vi "Find New Corners.vi"(0 "Updated Map":T1, 1 "Point":cluster{"Col":i16, "Row":i16}, 2 "# safety grids":i32=4) -> (5 "Corners":cluster{"Col":i16, "Row":i16}[](array[cluster]))   [LabVIEW 2009]
uses:
  <vilib>/Analysis/Matrix/Datatypes/RealMatrix.ctl
  <vilib>/Analysis/Matrix/NI_Matrix.lvlib
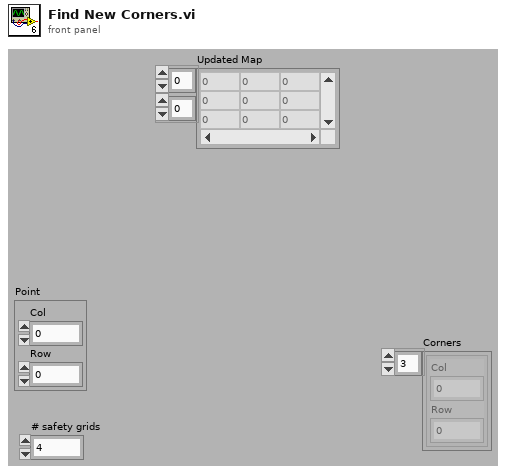
[diagram p1: front panel]
types:
  T1 = typedef "NI_Matrix.lvlib/RealMatrix.ctl" = dbl[][]
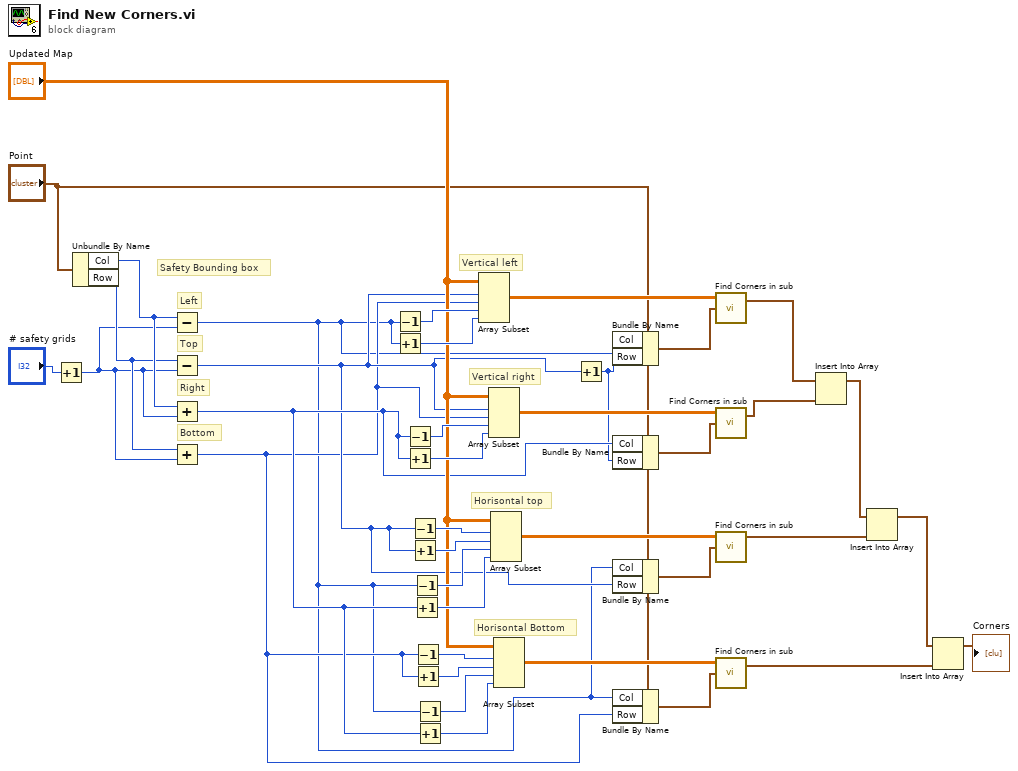
[diagram p0: block diagram]
diagram:
  # "Horisontal Bottom"
  # "Horisontal top"
  # "Vertical right"
  # "Vertical left"
  # "Safety Bounding box"
  # "Bottom"
  # "Top"
  # "Right"
  # "Left"
  n1 = Increment(x="# safety grids") -> (x+1=w2:i32)
  n2 = Unbundle By Name("Point") -> ("Col"=w38:i16, "Row"=w37:i16)
  n3 = Subtract(x=w38, y=w2) -> (x-y=w10:i32)
  n4 = Subtract(x=w37, y=w2) -> (x-y=w12:i32)
  n5 = Add(x=w38, y=w2) -> (x+y=w14:i32)
  n6 = Add(x=w37, y=w2) -> (x+y=w11:i32)
  n7 = Decrement(x=w10) -> (x-1=w36:i32)
  n8 = Increment(x=w10) -> (x+1=w35:i32)
  n9 = Decrement(x=w14) -> (x-1=w33:i32)
  n10 = Increment(x=w14) -> (x+1=w32:i32)
  n11 = Decrement(x=w12) -> (x-1=w29:i32)
  n12 = Increment(x=w12) -> (x+1=w28:i32)
  n13 = Decrement(x=w10) -> (x-1=w27:i32)
  n14 = Increment(x=w14) -> (x+1=w26:i32)
  n15 = Decrement(x=w11) -> (x-1=w24:i32)
  n16 = Increment(x=w11) -> (x+1=w23:i32)
  n17 = Decrement(x=w10) -> (x-1=w22:i32)
  n18 = Increment(x=w14) -> (x+1=w21:i32)
  n19 = Array Subset(array="Updated Map", index (row)=w12, length (row)=w11, index (col)=w36, length (col)=w35) -> (w34:T1)
  n20 = Array Subset(array="Updated Map", index (row)=w12, length (row)=w11, index (col)=w33, length (col)=w32) -> (w31:T1)
  n21 = Array Subset(array="Updated Map", index (row)=w29, length (row)=w28, index (col)=w27, length (col)=w26) -> (w30:T1)
  n22 = Array Subset(array="Updated Map", index (row)=w24, length (row)=w23, index (col)=w22, length (col)=w21) -> (w25:T1)
  n23 = Increment(x=w12) -> (x+1=w13:i32)
  n24 = Bundle By Name(cluster="Point", "Col"=w10, "Row"=w13) -> (w19:cluster{"Col":i16, "Row":i16})
  n25 = Bundle By Name(cluster="Point", "Col"=w14, "Row"=w13) -> (w18:cluster{"Col":i16, "Row":i16})
  n26 = Bundle By Name(cluster="Point", "Col"=w10, "Row"=w12) -> (w17:cluster{"Col":i16, "Row":i16})
  n27 = Bundle By Name(cluster="Point", "Col"=w10, "Row"=w11) -> (w16:cluster{"Col":i16, "Row":i16})
  n28 = call "Find Corners in sub.vi"("Start point"=w19, "Sub Matrix\n(Object edge)"=w34) -> ("Corners"=w9:cluster{"X":i16, "Y":i16}[])  [unwired: 2 in]
  n29 = call "Find Corners in sub.vi"("Start point"=w18, "Sub Matrix\n(Object edge)"=w31) -> ("Corners"=w8:cluster{"X":i16, "Y":i16}[])  [unwired: 2 in]
  n30 = call "Find Corners in sub.vi"("Start point"=w17, "Sub Matrix\n(Object edge)"=w30) -> ("Corners"=w6:cluster{"X":i16, "Y":i16}[])  [unwired: 2 in]
  n31 = call "Find Corners in sub.vi"("Start point"=w16, "Sub Matrix\n(Object edge)"=w25) -> ("Corners"=w4:cluster{"X":i16, "Y":i16}[])  [unwired: 2 in]
  n32 = Insert Into Array(array=w9, new element=w8) -> (w7:cluster{"X":i16, "Y":i16}[])  [unwired: 1 in]
  n33 = Insert Into Array(array=w7, new element=w6) -> (w5:cluster{"X":i16, "Y":i16}[])  [unwired: 1 in]
  n34 = Insert Into Array(array=w5, new element=w4) -> (→"Corners":cluster{"X":i16, "Y":i16}[])  [unwired: 1 in]
